vi "_Analyze Old HTML.vi"(0 "HTML File Path":path, 11 "error in":errorcluster) -> (4 "HTML File Path out":path, 8 "Info extracted from old HTML":T1={"_vi_name_"="", "_vi_description_text_"="", "_vi_controls_and_indicators_descriptions_"="", "_name_of_owning_library_"="", "_owning_library_html_"="", "_Packages_"="Base Package", "_Platforms_"="Windows", "_details_text_"="Put details here", "_example_screenshot_"="", "_example_vi_"="", "_path_to_example_file_"=path "", "IsDetailsON?"=FALSE, "IsOwningLibraryON?"=FALSE, "IsExamplesON?"=FALSE, "IsTableON?"=FALSE, "IsScrollableON?"=FALSE, "IsDetailedHelpLinkON?"=FALSE, "Table Objects array"=[], "Table Descriptions array"=[], "Table Links array"=[], "Start path location"=enum."VI folder"}, 15 "error out":errorcluster)   [LabVIEW 2012]
uses:
  _Controls and TypeDefs/InfoFromOldHTML_cluster.ctl
  _Controls and TypeDefs/StartPathLocation_enum.ctl
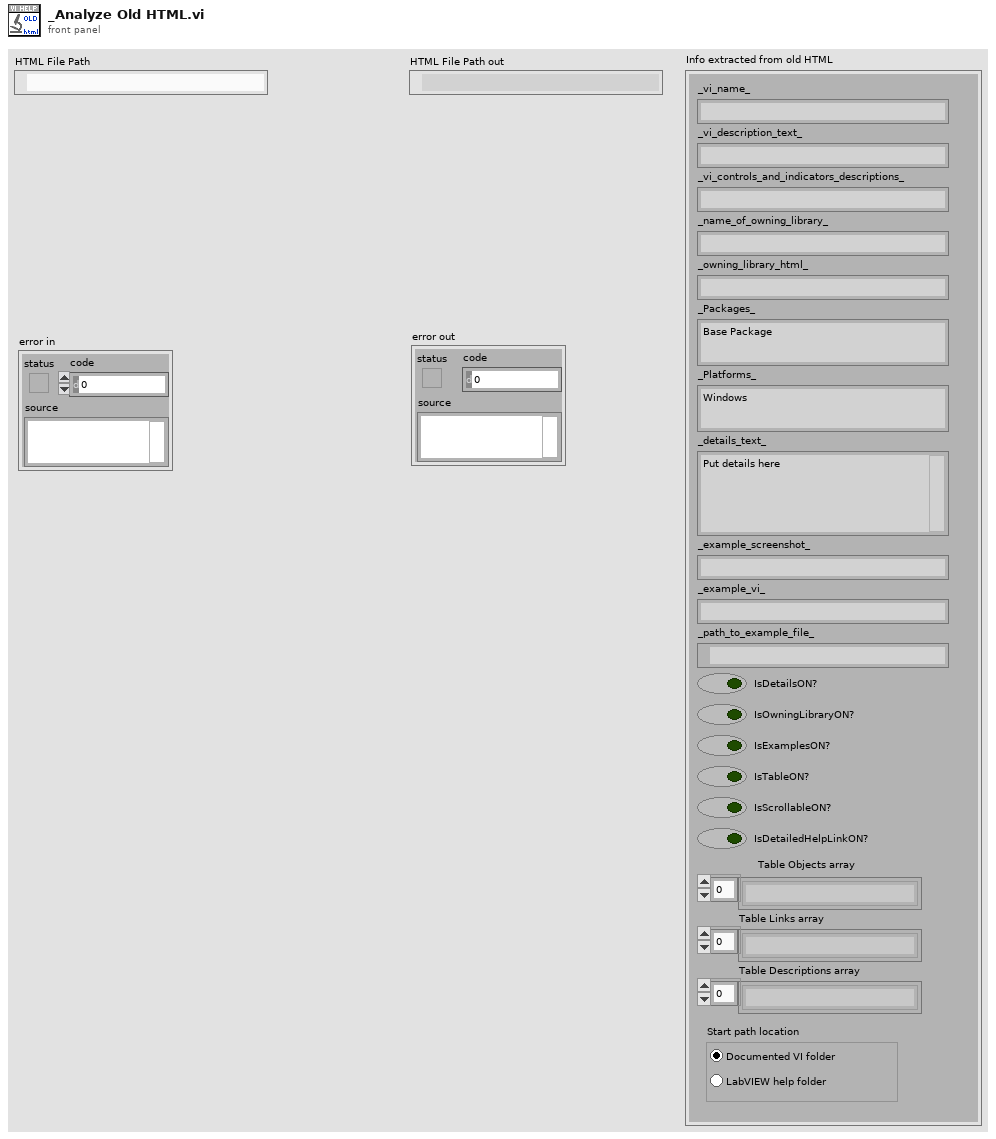
[diagram p1: front panel]
types:
  T1 = typedef "InfoFromOldHTML_cluster.ctl" = cluster{"_vi_name_":string, "_vi_description_text_":string, "_vi_controls_and_indicators_descriptions_":string, "_name_of_owning_library_":string, "_owning_library_html_":string, "_Packages_":string, "_Platforms_":string, "_details_text_":string, "_example_screenshot_":string, "_example_vi_":string, "_path_to_example_file_":path, "IsDetailsON?":bool, "IsOwningLibraryON?":bool, "IsExamplesON?":bool, "IsTableON?":bool, "IsScrollableON?":bool, "IsDetailedHelpLinkON?":bool, "Table Objects array":string[], "Table Descriptions array":string[], "Table Links array":string[], "Start path location":T2}
  T2 = typedef "StartPathLocation_enum.ctl" = enum32{"VI folder", "Help folder"}
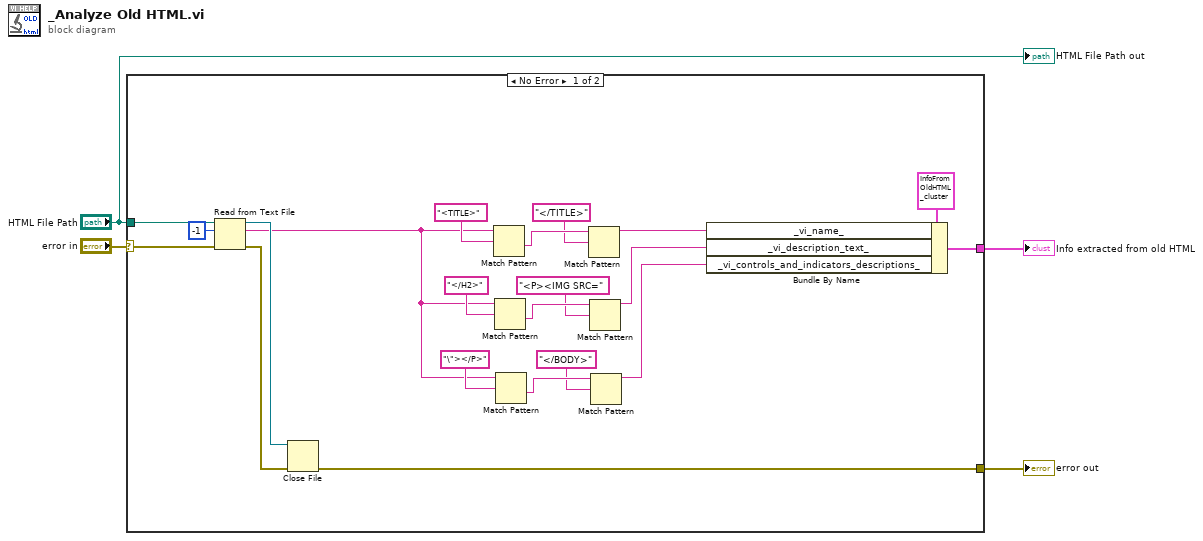
[diagram p0: block diagram]
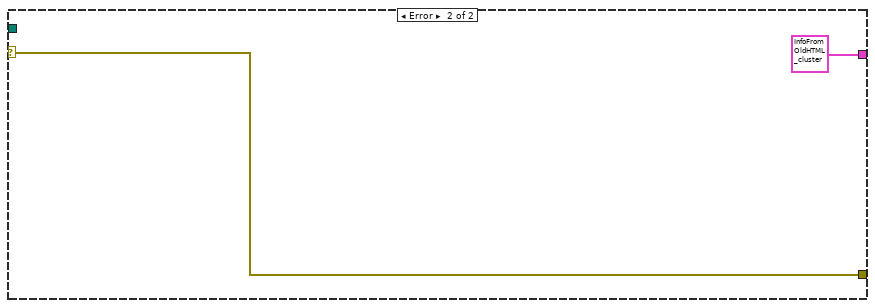
[diagram p2: hidden frame]
diagram:
  n1 = case shown="No Error" "error in" {
    selector: "error in" -> [w5 w27]
    tunnel: "HTML File Path" -> [w22 _]
    tunnel: [w17 T1 {"_vi_name_"="", "_vi_description_text_"="", "_vi_controls_and_indicators_descriptions_"="", "_name_of_owning_library_"="", "_owning_library_html_"="", "_Packages_"="Base Package", "_Platforms_"="Windows", "_details_text_"="Put details here", "_example_screenshot_"="", "_example_vi_"="", "_path_to_example_file_"=path "", "IsDetailsON?"=FALSE, "IsOwningLibraryON?"=FALSE, "IsExamplesON?"=FALSE, "IsTableON?"=FALSE, "IsScrollableON?"=FALSE, "IsDetailedHelpLinkON?"=FALSE, "Table Objects array"=[], "Table Descriptions array"=[], "Table Links array"=[], "Start path location"=enum."VI folder"} ("Info extracted from old HTML")] -> w4
    tunnel: [w15 w27] -> w3
    frame No Error {
      n2 = Read from Text File(file (use dialog)=w22, count=-1, error in=w5) -> (refnum out=w23:refnum<file>, text=w8:string, error out=w24:errorcluster)  [unwired: 1 in, 1 out]
      n3 = Close File(refnum=w23, error in=w24) -> (error out=w15:errorcluster)  [unwired: 1 out]
      n4 = Match Pattern(string=w8, regular expression="<TITLE>" ("search string")) -> (after substring=w20:string)  [unwired: 1 in, 3 out]
      n5 = Match Pattern(string=w8, regular expression="</H2>" ("search string")) -> (after substring=w13:string)  [unwired: 1 in, 3 out]
      n6 = Match Pattern(string=w8, regular expression="\"></P>" ("search string")) -> (after substring=w10:string)  [unwired: 1 in, 3 out]
      n7 = Match Pattern(string=w20, regular expression="</TITLE>") -> (before substring=w16:string)  [unwired: 1 in, 3 out]
      n8 = Match Pattern(string=w13, regular expression="<P><IMG SRC=") -> (before substring=w7:string)  [unwired: 1 in, 3 out]
      n9 = Match Pattern(string=w10, regular expression="</BODY>") -> (before substring=w6:string)  [unwired: 1 in, 3 out]
      n10 = Bundle By Name(cluster=T1 {"_vi_name_"="", "_vi_description_text_"="", "_vi_controls_and_indicators_descriptions_"="", "_name_of_owning_library_"="", "_owning_library_html_"="", "_Packages_"="", "_Platforms_"="", "_details_text_"="", "_example_screenshot_"="", "_example_vi_"="", "_path_to_example_file_"=path "", "IsDetailsON?"=FALSE, "IsOwningLibraryON?"=FALSE, "IsExamplesON?"=FALSE, "IsTableON?"=FALSE, "IsScrollableON?"=FALSE, "IsDetailedHelpLinkON?"=FALSE, "Table Objects array"=[], "Table Descriptions array"=[], "Table Links array"=[], "Start path location"=enum."VI folder"} ("Info extracted from old HTML"), "_vi_name_"=w16, "_vi_description_text_"=w7, "_vi_controls_and_indicators_descriptions_"=w6) -> (w17:T1)
    }
    frame Error {
    }
  }
  "error out" <- w3
  "Info extracted from old HTML" <- w4
  "HTML File Path out" <- "HTML File Path"
